vi "add node name.vi"(8 "error in (no error)":errorcluster, 11 "dvr in":refnum<data-value>) -> (0 "error out":errorcluster, 3 "dvr out":refnum<data-value>)   [LabVIEW 2020, in "Publisher Subscriber.lvlib"]
uses:
  Publisher Subscriber.lvlib
  Controls/data cluster.ctl
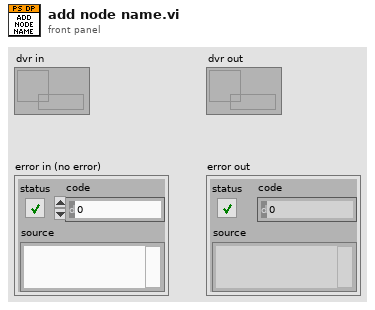
[diagram p1: front panel]
types:
  T1 = cluster{"queue ref":refnum<queue>, "subscription map ref":refnum<data-value>, "Command":string, "Data":variant, "Subscriptions []":set{string}, "variable dvr refs":refnum<data-value>}
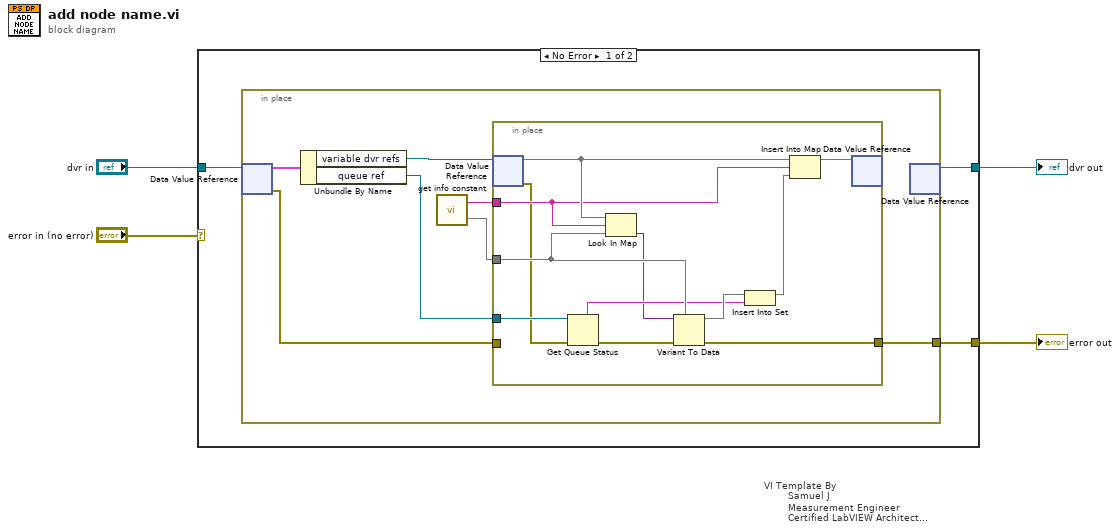
[diagram p0: block diagram]
diagram:
  n1 = case "VI Template By\n        Samuel J\n        Measurement Engineer\n        Certified LabVIEW Architect\n        Vestas Technology R&D Chennai" shown="No Error" "error in (no error)" {
    selector: "error in (no error)" -> [_ w27]
    tunnel: "dvr in" -> [w7 w28]
    tunnel: [w6 w28] -> w2
    tunnel: [w5 w27] -> w4
    frame No Error {
      n2 = in-place {
        in-place-border: [w10] -> w5
        n3 = in-place-dvr #1(w7) -> (w14:T1, w9:errorcluster)
        n4 = Unbundle By Name(w14) -> ("variable dvr refs"=w13:refnum<data-value>, "queue ref"=w8:refnum<queue>)
        n5 = call "get info constant.vi"() -> ("set"=w11:set{string}, "String"=w12:string)  [unwired: 4 in]
        n6 = in-place {
          in-place-border: w12 -> [w23]
          in-place-border: w11 -> [w21]
          in-place-border: w8 -> [w18]
          in-place-border: w9 -> [_]
          in-place-border: [w15] -> w10
          n7 = in-place-dvr #2(w13) -> (w26:map{string, variant}, w17:errorcluster)
          n8 = Get Queue Status(queue=w18, error in (no error)=w17) -> (queue name=w20:string, error out=w16:errorcluster)  [unwired: 1 in, 6 out]
          n9 = Look In Map(map=w26, key=w23, default value=w21) -> (value=w19:variant)  [unwired: 1 out]
          n10 = Variant To Data(error in=w16, type=w21, Variant=w19) -> (data=w25:set{string}, error out=w15:errorcluster)
          n11 = Insert Into Set(10:w20, 11:w25) -> (3:w24:set{string})  [unwired: 1 out]
          n12 = Insert Into Map(map in=w26, key=w23, value=w24) -> (map out=w22:map{string, variant})  [unwired: 2 out]
          n13 = in-place-dvr #2(w22) -> ()  [unwired: 2 out]
        }
        n14 = in-place-dvr #1() -> (w6:refnum<data-value>)  [unwired: 1 in, 1 out]
      }
    }
    frame Error {
    }
  }
  "error out" <- w4
  "dvr out" <- w2
